vi "Main.vi"() -> ()   [LabVIEW 2017]
uses:
  Presentation/Page-XControl/Page-XControl.xctl
  0b84e2c4-0d44-4a77-8dcb-aa425a784c0e.vi
  Presentation/Slide/Slide.lvclass
panel:
  in  "Open":bool
  out "PageXCtrl":u32(xcontrol)
  in  "Stop":bool
  in  "Last":bool
  in  "First":bool
  in  "Left":bool
  in  "Right":bool
  out "LowerLeft":string caption="String"
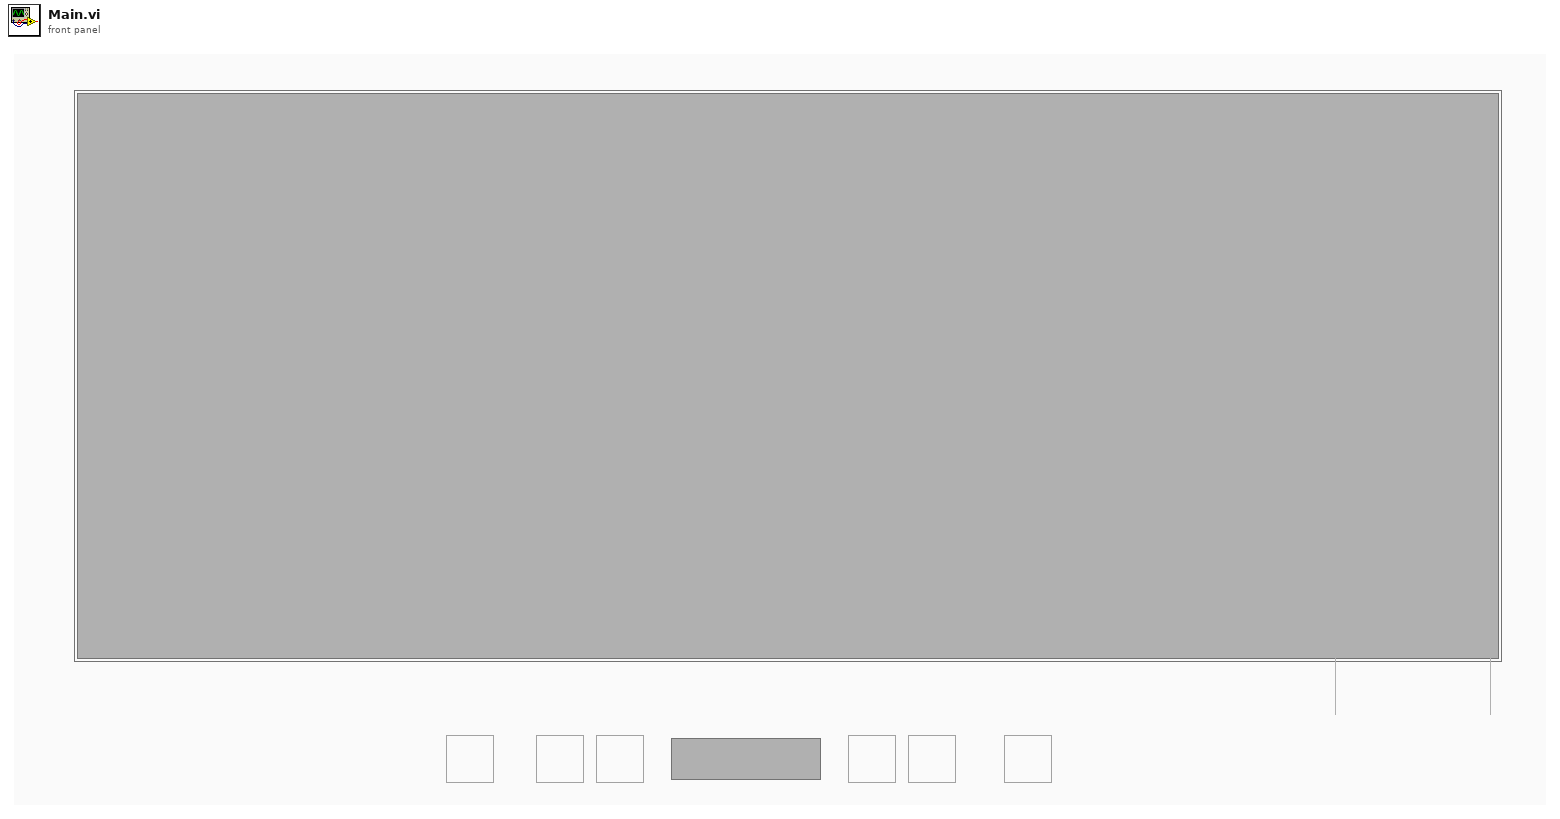
[diagram p1: front panel]
types:
  T1 = typedef "eventvkey.ctl" = enum16{"ASCII", "Enter", "Return", "Shift", "Ctrl", "Alt", "Cmd", "Opt", "Caps", "NumLock", "Clear", "Break", "Up", "Down", "Left", "Right", "Insert", "Delete", "Home", "End", "PageUp", "PageDown", "Escape", "Help", "Pause", "ScrollLock", "F1", "F2", "F3", "F4", "F5", "F6", "F7", "F8", "F9", "F10", "F11", "F12", "F13", "F14", "F15", "F16", "F17", "F18", "F19", "F20", "F21", "F22", "F23", "F24", "Play", "VolumeUp", "VolumeDown", "Mute", "Two Byte Char"}
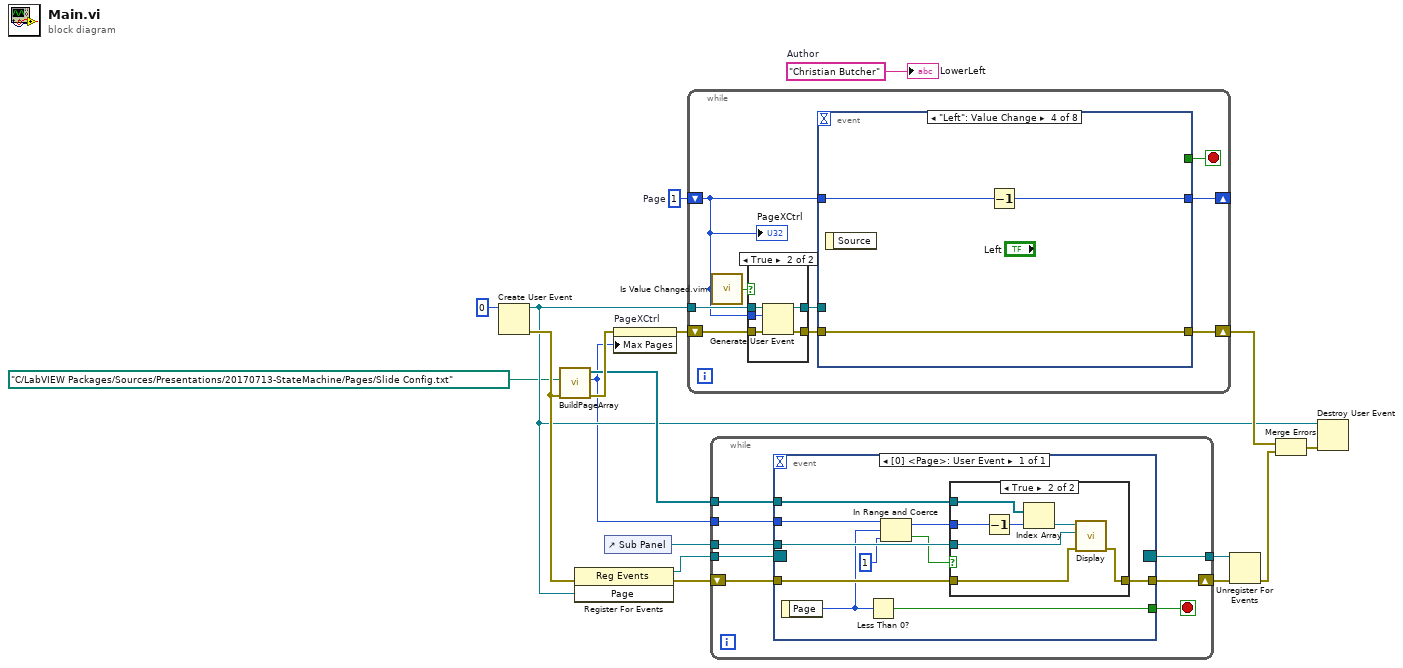
[diagram p0: block diagram]
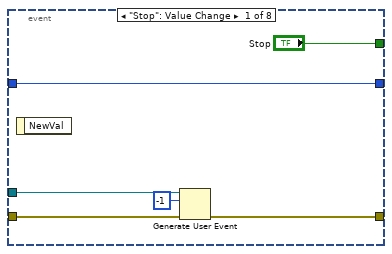
[diagram p4: hidden frame]
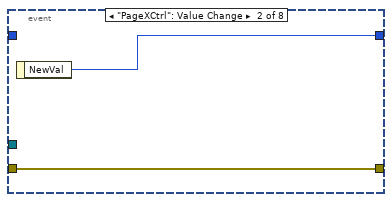
[diagram p5: hidden frame]
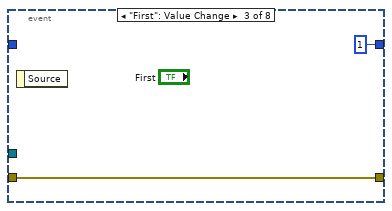
[diagram p6: hidden frame]
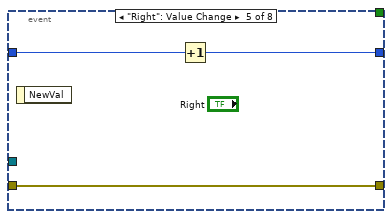
[diagram p7: hidden frame]
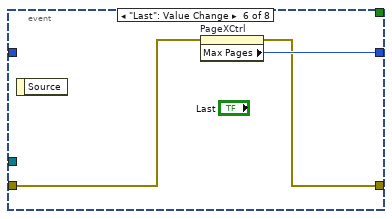
[diagram p8: hidden frame]
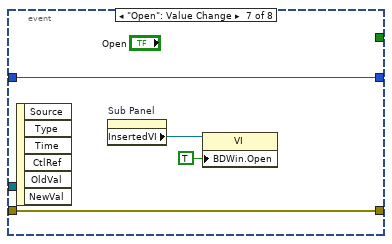
[diagram p9: hidden frame]
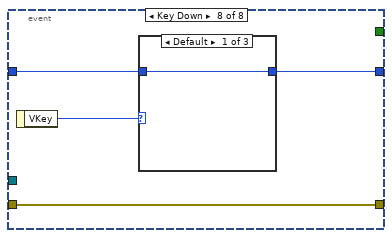
[diagram p10: hidden frame]
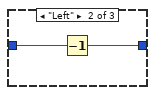
[diagram p11: hidden frame]
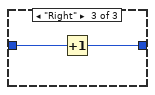
[diagram p12: hidden frame]
diagram:
  w16 = "Christian Butcher"  # Author
  w17 = u32 1  # Page
  n1 = Create User Event(user event datatype=0 ("Page")) -> (user event=w4:refnum<user-event>, error out=w13:errorcluster)  [unwired: 1 in]
  n2 = call "BuildPageArray.vi"("error in (no error)"=w13, "Config File Path"=path "C:/LabVIEW Packages/Sources/Presentations/20170713-StateMachine/Pages/Slide Config.txt") -> ("error out"=w18:errorcluster, "Num Pages"=w1:i32, "Array"=w10:refnum<class "Slide.lvclass">[])  [unwired: 7 in]
  n3 = register-events(error in=w13, w4) -> (reference out=w11:refnum<event-registration>, error out=w12:errorcluster)  [unwired: 1 in]
  n4 = control-ref of="Sub Panel"() -> (w2:refnum<vi>)
  n5 = property on="PageXCtrl" class="Page-XControl (strict)"(error in=w18, "Max Pages"=w1) -> (error out=w15:errorcluster)  [unwired: 1 in, 1 out]
  n6 = while {
    shift-right: [w26] -> _
    shift-left: w17 -> [w20]
    shift-right: [w24] -> w7
    shift-left: w15 -> [w25]
    tunnel: w4 -> [w22]
    stop <- w27 stop-if-true
    n7 = call "Is Value Changed.vim"("value"=w20) -> ("changed or first call?"=w19:bool)
    n8 = case shown="True" w19 {
      tunnel: w25 -> [w28 w34]
      tunnel: [w28 w33] -> w23
      tunnel: w22 -> [w29 w32]
      tunnel: w20 -> [_ w31]
      tunnel: [w29 w30] -> w21
      frame False {
      }
      frame True {
        n9 = Generate User Event(user event=w32, event data cluster=w31, error in=w34) -> (user event out=w30:refnum<user-event>, error out=w33:errorcluster)  [unwired: 1 in]
      }
    }
    n10 = event shown="[3] \"Left\": Value Change" {
      selector: _ -> [_ _ _ _ _ _ _ _]
      dyn-events: _ -> [_ _ _ _ _ _ _ _]
      timeout: _ -> [_ _ _ _ _ _ _ _]
      tunnel: ["Stop" _ _ _ _ _ _ _] -> w27
      tunnel: w20 -> [w40 _ _ w47 w50 _ w57 w59]
      tunnel: [w40 w41 u32 1 ("NewVal") w46 w49 w53 w57 w58] -> w26
      tunnel: w23 -> [w38 w42 w44 w45 w48 w52 w56 w61]
      tunnel: [w37 w42 w44 w45 w48 w51 w56 w61] -> w24
      tunnel: w21 -> [w36 _ _ _ _ _ _ _]
      event "Stop": Value Change {
        n11 = event-data() -> ()  [unwired: 1 in, 1 out]
        n12 = Generate User Event(user event=w36, event data cluster=-1 ("event data"), error in=w38) -> (error out=w37:errorcluster)  [unwired: 1 in, 1 out]
      }
      event "PageXCtrl": Value Change {
        n13 = event-data() -> ("NewVal"=w41:u32)  [unwired: 1 in]
      }
      event "First": Value Change {
        n14 = event-data() -> ()  [unwired: 1 in, 1 out]
      }
      event "Left": Value Change {
        n15 = event-data() -> ()  [unwired: 1 in, 1 out]
        n16 = Decrement(x=w47) -> (x-1=w46:u32)
      }
      event "Right": Value Change {
        n17 = event-data() -> ()  [unwired: 1 in, 1 out]
        n18 = Increment(x=w50) -> (x+1=w49:u32)
      }
      event "Last": Value Change {
        n19 = event-data() -> ()  [unwired: 1 in, 1 out]
        n20 = property on="PageXCtrl" class="Page-XControl (strict)"(error in=w52) -> (error out=w51:errorcluster, "Max Pages"=w53:u32)  [unwired: 1 in, 1 out]
      }
      event "Open": Value Change {
        n21 = event-data() -> ()  [unwired: 1 in, 6 out]
        n22 = property on="Sub Panel" class="SubPnl"() -> ("InsertedVI"=w55:refnum<vi>)  [unwired: 2 in, 2 out]
        n23 = property on="Property Node" class="VI"(reference=w55, "BDWin.Open"=TRUE ("Block Diagram Window:Open")) -> ()  [unwired: 1 in, 2 out]
      }
      event Key Down {
        n24 = event-data() -> ("VKey"=w60:T1)  [unwired: 1 in]
        n25 = case shown="Default" w60 {
          tunnel: w59 -> [w62 w64 w66]
          tunnel: [w62 w63 w65] -> w58
          frame Default {
          }
          frame "Left" {
            n26 = Decrement(x=w64) -> (x-1=w63:u32)
          }
          frame "Right" {
            n27 = Increment(x=w66) -> (x+1=w65:u32)
          }
        }
      }
    }
    "PageXCtrl" <- w20
  }
  n28 = while {
    tunnel: w11 -> [w73]
    shift-right: [w70] -> w9
    shift-left: w12 -> [w74]
    tunnel: w10 -> [w71]
    tunnel: [w69] -> w8
    tunnel: w2 -> [w68]
    tunnel: w1 -> [w67]
    stop <- w72 stop-if-true
    n29 = event shown="[0] <Page>: User Event" {
      selector: w73 -> [_]
      dyn-events: [_] -> w69
      timeout: _ -> [_]
      tunnel: w74 -> [w81]
      tunnel: [w84] -> w72
      tunnel: w71 -> [w83]
      tunnel: [w80] -> w70
      tunnel: w68 -> [w82]
      tunnel: w67 -> [w79]
      event User Event {
        n30 = event-data() -> ("Page"=w78:i32)  [unwired: 1 in]
        n31 = Less Than 0?(x=w78) -> (x < 0?=w84:bool)
        n32 = In Range and Coerce(upper limit=w79, x=w78, lower limit=u32 1) -> (coerced(x)=w77:u32, In Range?=w75:bool)
        n33 = case shown="True" w75 {
          tunnel: w83 -> [_ w92]
          tunnel: w82 -> [_ w91]
          tunnel: w81 -> [w85 w90]
          tunnel: [w85 w89] -> w80
          tunnel: w77 -> [_ w88]
          frame False {
          }
          frame True {
            n34 = Decrement(x=w88) -> (x-1=w86:u32)
            n35 = Index Array(array=w92, index=w86) -> (element=w87:refnum<class "Slide.lvclass">)
            n36 = call-dynamic "Display.vi"("error in (no error)"=w90, "SubPnl Refnum"=w91, "Slide in"=w87) -> ("error out"=w89:errorcluster)  [unwired: 7 in, 1 out]
          }
        }
      }
    }
  }
  n37 = Unregister For Events(event registration refnum=w8, error in=w9) -> (error out=w6:errorcluster)
  n38 = Merge Errors(w7, w6) -> (w5:errorcluster)
  n39 = Destroy User Event(user event=w4, error in=w5) -> ()  [unwired: 1 out]
  "LowerLeft" <- w16
